vi "定时启动 (子VI).vi"   [LabVIEW 2016, in "CODCr库.lvlib"]
types:
  T1 = enum16{"启动测量", "标样核查", "零点核查", "跨度核查", "空白测试", "平行样测试", "加标回收", "空白校准", "标样校准", "初始化（清洗）", "停止测试", "仪器重启", "校时", "模式设置", "测量间隔设置"}
  T2 = cluster{"测量模式":enum16{"水样测量", "标样核查", "零点核查", "跨度核查", "空白测试", "加标回收", "平行样", "校零", "校标"}}
  T3 = cluster{"控制命令":enum16{"启动测量", "标样核查", "零点核查", "跨度核查", "空白测试", "平行样测试", "加标回收", "空白校准", "标样校准", "初始化（清洗）", "停止测试", "仪器重启", "校时", "模式设置", "测量间隔设置"}, "周期设置类型":enum16{"定点启动", "间隔启动"}, "定时功能启用":bool, "定时间隔":dbl, "24H周期设置":bool[], "零点核查时间":u16, "跨度核查时间":u16, "质控频次":enum16{"关闭", "每天", "星期一", "星期二", "星期三", "星期四", "星期五", "星期六", "星期日"}}
  T4 = enum16{"关闭", "每天", "星期一", "星期二", "星期三", "星期四", "星期五", "星期六", "星期日"}
  T5 = typedef "LVDateTimeRec.ctl" = cluster{"秒数的小数部分":dbl, "秒":i32, "分":i32, "时":i32, "日":i32, "月":i32, "年":i32, "天数（周）":i32, "天数（年）":i32, "DST":i32}
  T6 = cluster{"系统时间":timestamp, "工作状态":u16, "测量模式":u16, "告警代码":enum16{"无告警", "缺试剂告警", "缺水样告警", "缺蒸馏水告警", "缺标液告警", "仪表漏液告警", "标定异常告警", "超量程告警", "加热异常", "低试剂预警", "超上限告警", "超下限告警", "仪表内部其他异常", "滴定异常告警", "电极异常告警", "量程切换告警", "参数设置告警", "PH电极电位异常", "电导率电极异常", "浊度光度异常", "溶解氧电极异常", "溶解氧光强异常", "温度异常告警", "PH异常告警", "溶解氧异常告警", "电导率异常告警", "浊度异常告警", "叶绿素异常告警", "藻密度异常告警", "蓝绿藻异常告警", "ORP异常告警", "氨氮异常告警", "清洁刷异常告警", "SD卡异常告警", "蓝牙异常告警", "Wifi异常告警", "流程异常告警"}, "故障代码":enum16{"无故障", "电机故障", "温度故障", "通讯故障", "滴定故障"}, "日志代码":u16, "软件版本":u16, "F0":sgl, "F1":sgl, "F2":sgl, "F3":sgl, "T":sgl, "H":sgl, "id":u16, "flowid":u16, "量程":u16}
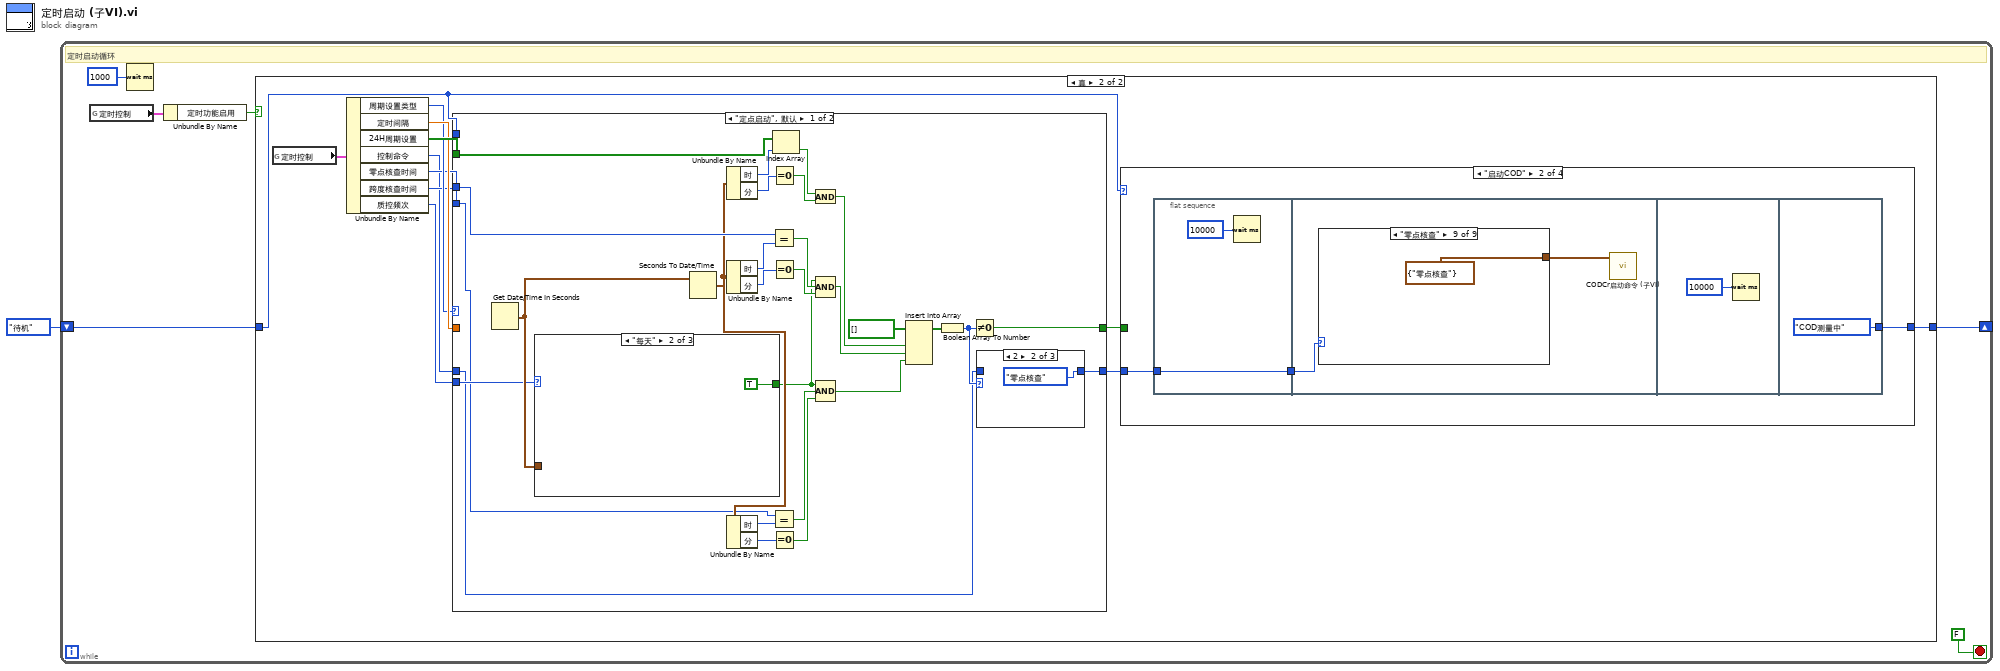
[diagram p0: block diagram]
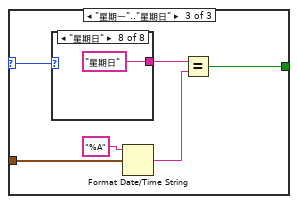
[diagram p4: hidden frame]
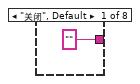
[diagram p5: hidden frame]
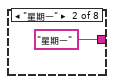
[diagram p6: hidden frame]
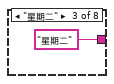
[diagram p7: hidden frame]
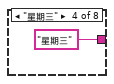
[diagram p8: hidden frame]
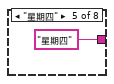
[diagram p9: hidden frame]
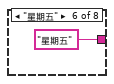
[diagram p10: hidden frame]
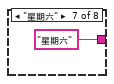
[diagram p11: hidden frame]
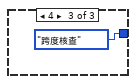
[diagram p13: hidden frame]
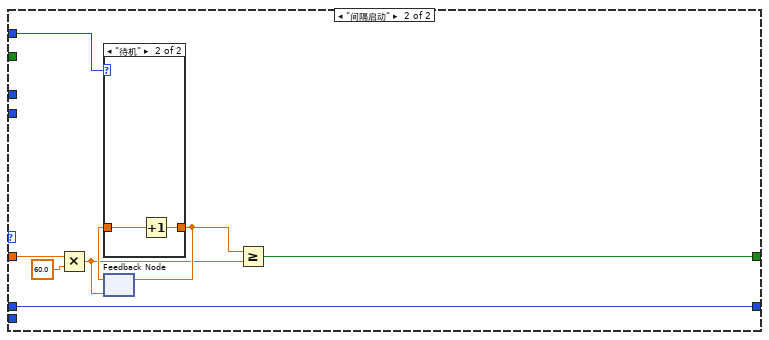
[diagram p14: hidden frame]
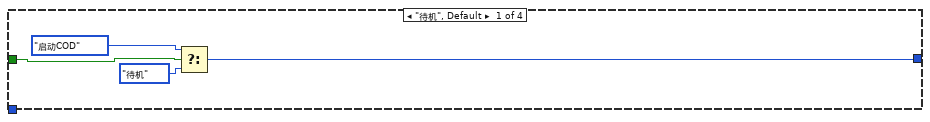
[diagram p16: hidden frame]
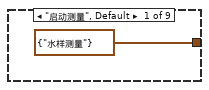
[diagram p17: hidden frame]
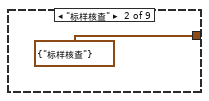
[diagram p18: hidden frame]
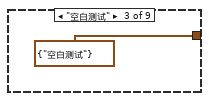
[diagram p19: hidden frame]
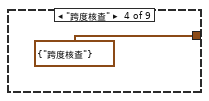
[diagram p20: hidden frame]
diagram:
  n1 = while {
    shift-right: [w6] -> _
    shift-left: enum16{"待机", "启动COD", "COD测量中", "延时"}."待机" -> [w5]
    stop <- FALSE stop-if-true
    # "定时启动循环"
    n2 = global read "CODcr全局变量.vi" "定时控制"() -> (w4:T3)
    n3 = Wait (ms)(milliseconds to wait=u32 1000 ("等待时间（毫秒）")) -> ()  [unwired: 1 out]
    n4 = Unbundle By Name(w4) -> ("定时功能启用"=w3:bool)
    n5 = case shown="真" w3 {
      tunnel: [w8 w20] -> w6
      tunnel: w5 -> [w8 w19]
      frame False {
      }
      frame True {
        n6 = global read "CODcr全局变量.vi" "定时控制"() -> (w13:T3)
        n7 = Unbundle By Name(w13) -> ("周期设置类型"=w14:enum16{"定点启动", "间隔启动"}, "定时间隔"=w15:dbl, "24H周期设置"=w16:bool[], "控制命令"=w9:T1, "零点核查时间"=w12:u16, "跨度核查时间"=w10:u16, "质控频次"=w11:T4)
        n8 = case shown="\"定点启动\", 默认" w14 {
          tunnel: w15 -> [_ w71]
          tunnel: w16 -> [w48 _]
          tunnel: w19 -> [_ w74]
          tunnel: [w24 w69] -> w18
          tunnel: w12 -> [w47 _]
          tunnel: w11 -> [w25 _]
          tunnel: w10 -> [w23 _]
          tunnel: w9 -> [w22 w67]
          tunnel: [w21 w67] -> w17
          frame "定点启动", Default {
            n9 = Get Date/Time In Seconds() -> (seconds since 1Jan1904=w43:timestamp)
            n10 = case shown="\"每天\"" w25 {
              selector: w25 -> [_ _ w53]
              tunnel: w43 -> [_ _ w54]
              tunnel: [_ TRUE w50] -> w32
              frame "关闭", Default {
              }
              frame "每天" {
              }
              frame "星期一".."星期日" {
                n11 = case shown="\"星期日\"" w53 {
                  tunnel: ["" ("时间格式字符串(%c)") "星期一" ("时间格式字符串(%c)") "星期二" ("时间格式字符串(%c)") "星期三" ("时间格式字符串(%c)") "星期四" ("时间格式字符串(%c)") "星期五" ("时间格式字符串(%c)") "星期六" ("时间格式字符串(%c)") "星期日" ("时间格式字符串(%c)")] -> w52
                  frame "关闭", Default {
                  }
                  frame "星期一" {
                  }
                  frame "星期二" {
                  }
                  frame "星期三" {
                  }
                  frame "星期四" {
                  }
                  frame "星期五" {
                  }
                  frame "星期六" {
                  }
                  frame "星期日" {
                  }
                }
                n12 = Format Date/Time String(time format string (%c)="%A" ("时间格式字符串(%c)"), seconds (now)=w54) -> (date/time string=w51:string)  [unwired: 1 in]
                n13 = Equal?(x=w52, y=w51) -> (x = y?=w50:bool)
              }
            }
            n14 = Seconds To Date/Time(time stamp (now)=w43) -> (date time rec=w33:T5)  [unwired: 1 in]
            n15 = Unbundle By Name(w33) -> ("时"=w46:i32, "分"=w45:i32)
            n16 = Unbundle By Name(w33) -> ("时"=w40:i32, "分"=w41:i32)
            n17 = Unbundle By Name(w33) -> ("时"=w35:i32, "分"=w34:i32)
            n18 = Equal?(x=w47, y=w40) -> (x = y?=w39:bool)
            n19 = Equal?(x=w23, y=w35) -> (x = y?=w36:bool)
            n20 = Equal To 0?(x=w45) -> (x = 0?=w44:bool)
            n21 = Equal To 0?(x=w41) -> (x = 0?=w38:bool)
            n22 = Equal To 0?(x=w34) -> (x = 0?=w37:bool)
            n23 = Index Array(array=w48, index=w46) -> (element=w42:bool)
            n24 = Compound Arithmetic op=AND ("复合运算")(w42, w44) -> (w30:bool)
            n25 = Compound Arithmetic op=AND ("复合运算")(w32, w39, w38) -> (w29:bool)
            n26 = Compound Arithmetic op=AND ("复合运算")(w32, w36, w37) -> (w28:bool)
            n27 = Insert Into Array(array=bool[] [], new element #1=w30, new element #2=w29, new element #3=w28) -> (w27:bool[])  [unwired: 1 in]
            n28 = Boolean Array To Number(Boolean array=w27) -> (number=w26:u32)
            n29 = Not Equal To 0?(x=w26) -> (x != 0?=w24:bool)
            n30 = case shown="2" w26 {
              tunnel: [w64 T1."零点核查" ("控制命令") T1."跨度核查" ("控制命令")] -> w21
              tunnel: w22 -> [w64 _ _]
              frame 0, Default {
              }
              frame 2 {
              }
              frame 4 {
              }
            }
          }
          frame "间隔启动" {
            n31 = Multiply(x=w71, y=60.0) -> (x*y=w68:dbl)
            n32 = feedback #1(w68) -> (w73:dbl)
            n33 = case shown="\"待机\"" w74 {
              tunnel: w73 -> [_ w76]
              tunnel: [_ w75] -> w72
              frame Default {
              }
              frame "待机" {
                n34 = Increment(x=w76) -> (x+1=w75:dbl)
              }
            }
            n35 = feedback-in #1(w72) -> ()
            n36 = Greater Or Equal?(x=w72, y=w68) -> (x >= y?=w69:bool)
          }
        }
        n37 = case shown="\"启动COD\"" w19 {
          tunnel: [w77 w83 w100 enum16{"待机", "启动COD", "COD测量中", "延时"}."待机"] -> w20
          tunnel: w18 -> [w80 _ _ _]
          tunnel: w17 -> [_ w81 _ _]
          frame "待机", Default {
            n38 = Select(t=enum16{"待机", "启动COD", "COD测量中", "延时"}."启动COD", s=w80, f=enum16{"待机", "启动COD", "COD测量中", "延时"}."待机") -> (s? t:f=w77:enum16{"待机", "启动COD", "COD测量中", "延时"})
          }
          frame "启动COD" {
            n39 = flat-sequence {
              tunnel: w81 -> [w85]
              tunnel: [w85] -> w82
              tunnel: w82 -> [w87]
              tunnel: [enum16{"待机", "启动COD", "COD测量中", "延时"}."COD测量中"] -> w83
              frame #0 {
                n40 = Wait (ms)(milliseconds to wait=u32 10000 ("等待时间（毫秒）")) -> ()  [unwired: 1 out]
              }
              frame #1 {
                n41 = case shown="\"零点核查\"" w87 {
                  tunnel: [T2 {"测量模式"=enum."水样测量"} ("启动测量模式") T2 {"测量模式"=enum."标样核查"} ("启动测量模式") T2 {"测量模式"=enum."空白测试"} ("启动测量模式") T2 {"测量模式"=enum."跨度核查"} ("启动测量模式") T2 {"测量模式"=enum."加标回收"} ("启动测量模式") T2 {"测量模式"=enum."平行样"} ("启动测量模式") T2 {"测量模式"=enum."校零"} ("启动测量模式") T2 {"测量模式"=enum."校标"} ("启动测量模式") T2 {"测量模式"=enum."零点核查"} ("启动测量模式")] -> w86
                  frame "启动测量", Default {
                  }
                  frame "标样核查" {
                  }
                  frame "空白测试" {
                  }
                  frame "跨度核查" {
                  }
                  frame "加标回收" {
                  }
                  frame "平行样测试" {
                  }
                  frame "空白校准" {
                  }
                  frame "标样校准" {
                  }
                  frame "零点核查" {
                  }
                }
                n42 = call "CODCr启动命令 (子VI).vi"("启动测量模式"=w86) -> ()  [unwired: 11 in]
              }
              frame #2 {
                n43 = Wait (ms)(milliseconds to wait=u32 10000 ("等待时间（毫秒）")) -> ()  [unwired: 1 out]
              }
              frame #3 {
              }
            }
          }
          frame "COD测量中" {
            n44 = flat-sequence {
              tunnel: [w105] -> w99
              tunnel: [w109] -> w100
              tunnel: w99 -> [w109]
              frame #0 {
                n45 = global read "CODcr全局变量.vi" "状态告警区"() -> (w102:T6)
                n46 = Unbundle By Name(w102) -> ("工作状态"=w103:u16)
                n47 = Equal?(x=w103, y=u16 0 ("工作状态")) -> (x = y?=w101:bool)
                n48 = Select(t=enum16{"待机", "启动COD", "COD测量中", "延时"}."延时", s=w101, f=enum16{"待机", "启动COD", "COD测量中", "延时"}."COD测量中") -> (s? t:f=w105:enum16{"待机", "启动COD", "COD测量中", "延时"})
              }
              frame #1 {
                n49 = Wait (ms)(milliseconds to wait=u32 5000 ("等待时间（毫秒）")) -> ()  [unwired: 1 out]
              }
            }
          }
          frame "延时" {
          }
        }
      }
    }
  }
